vi "Interfaz.vi"() -> ()   [LabVIEW 2025]
uses:
  <vilib>/httpClient/PUTBuffer.vi
  <vilib>/httpClient/LabVIEWHTTPClient.lvlib
panel:
  in  "Ganacias \ny \nSetpoint":T1
  in  "Paro":bool
  out "Error 2":dbl(graph)
  out "Fuera de servicio":bool
  out "Posicion":dbl
  out "Heartbeat":dbl
  out "error\n out":errorcluster
  out "Error":dbl
  # "INSTITUTO POLITECNICO NACIONAL"
  # "Unidad Profesional Interdisciplinaria de Ingeniería\nCampus Zacatecas"
  # "Botones"
  # "Resultados"
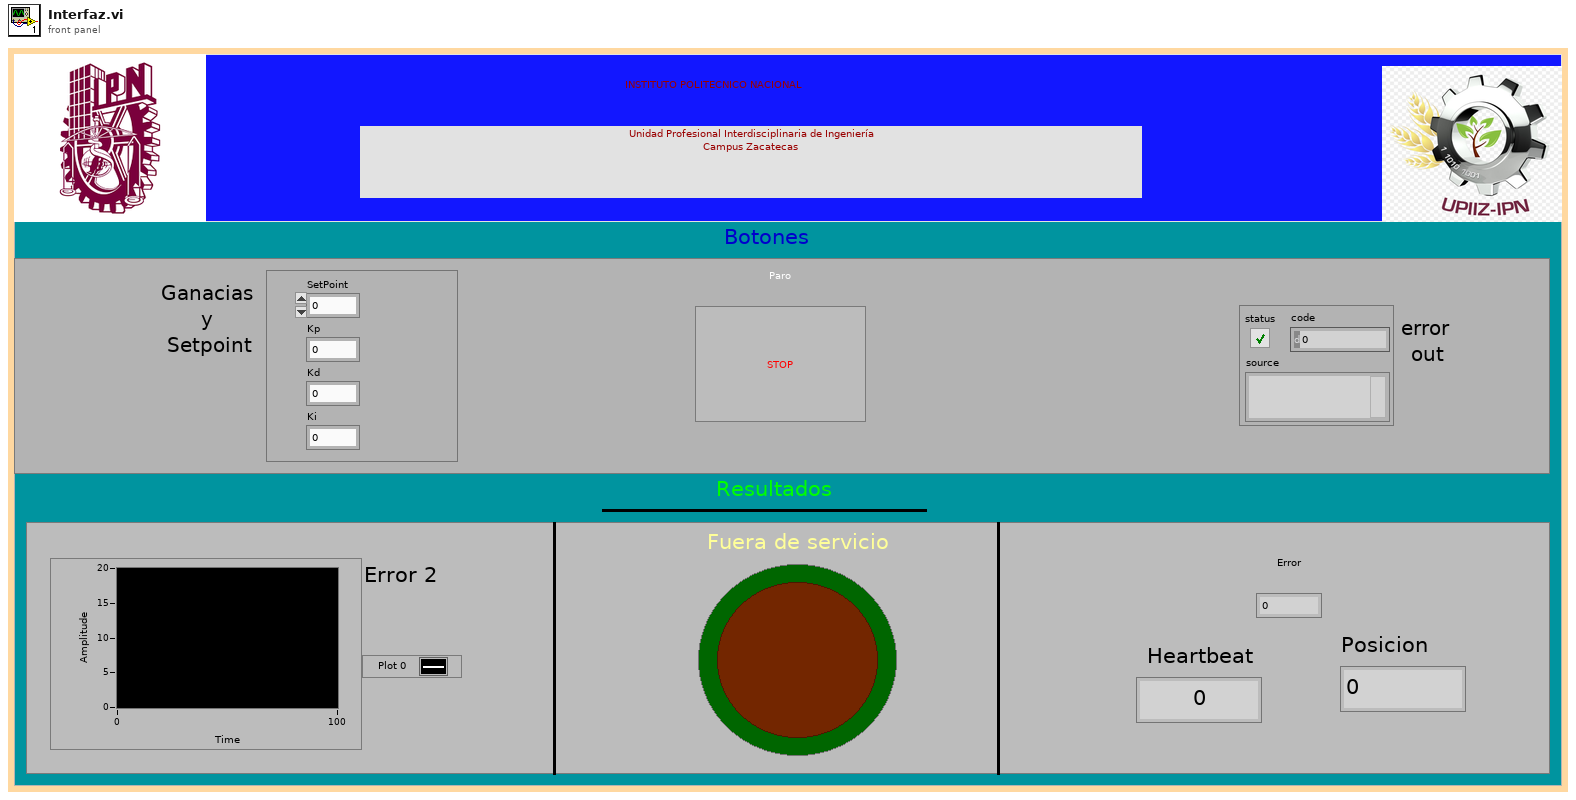
[diagram p1: front panel]
types:
  T1 = cluster{"SetPoint":dbl, "Kp":dbl, "Ki":dbl, "Kd":dbl}
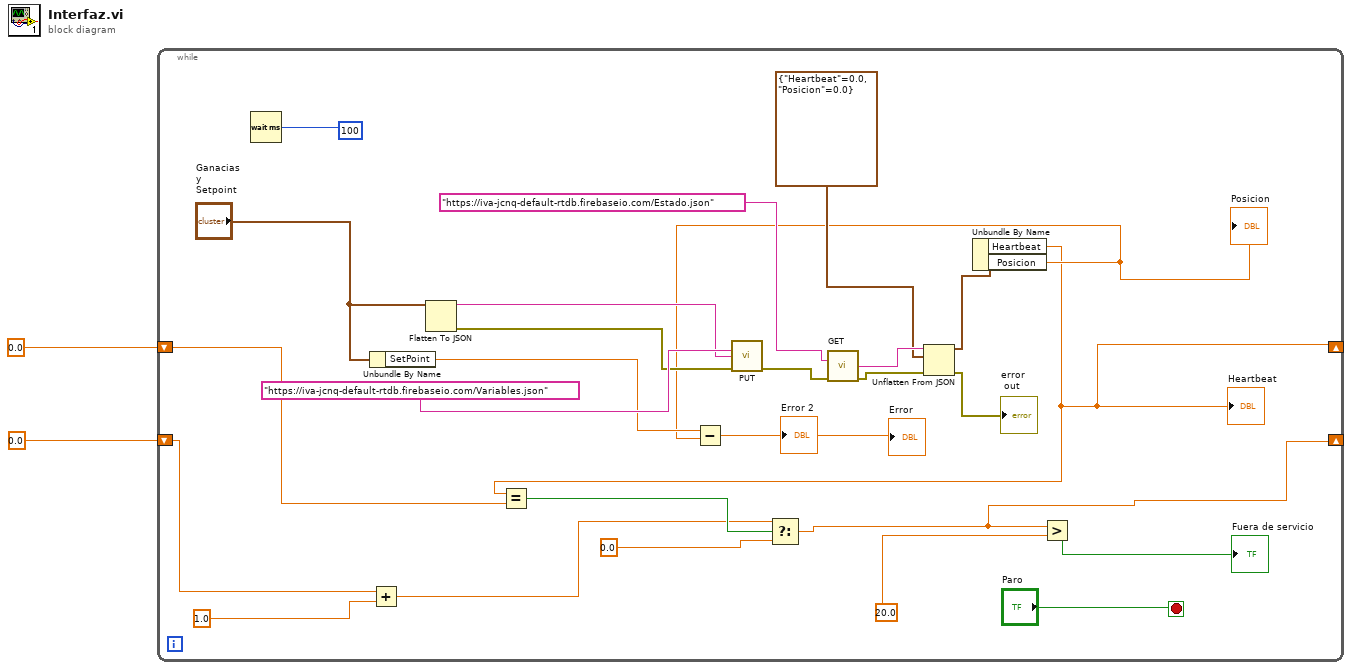
[diagram p0: block diagram]
diagram:
  n1 = while {
    shift-right: [w3] -> _
    shift-left: 0.0 ("x") -> [w17]
    shift-right: [w9] -> _
    shift-left: 0.0 ("x") -> [w14]
    stop <- "Paro" stop-if-true
    n2 = Wait (ms)(milliseconds to wait=u32 100) -> ()  [unwired: 1 out]
    n3 = Unbundle By Name("Ganacias \ny \nSetpoint") -> ("SetPoint"=w19:dbl)
    n4 = Add(x=w14, y=1.0) -> (x+y=w12:dbl)
    n5 = Flatten To JSON(anything="Ganacias \ny \nSetpoint") -> (JSON string=w25:string, 11:w26:errorcluster)  [unwired: 2 in]
    n6 = call-poly <vilib>:"PUT.vi"("url"="https://iva-jcnq-default-rtdb.firebaseio.com/Variables.json", "buffer"=w25, "error in (no error)"=w26) -> ("error out"=w24:errorcluster)  [unwired: 9 in, 3 out]
    n7 = call <vilib>:"GET.vi"("url"="https://iva-jcnq-default-rtdb.firebaseio.com/Estado.json", "error in (no error)"=w24) -> ("body"=w22:string, "error out"=w7:errorcluster)  [unwired: 10 in, 2 out]
    n8 = Unflatten From JSON(JSON string=w22, type and defaults=cluster{"Heartbeat":dbl, "Posicion":dbl} {"Heartbeat"=0.0, "Posicion"=0.0}, error in (no error)=w7) -> (value=w5:cluster{"Heartbeat":dbl, "Posicion":dbl}, error out=→"error\n out":errorcluster)  [unwired: 4 in]
    n9 = Unbundle By Name(w5) -> ("Heartbeat"=w3:dbl, "Posicion"=w4:dbl)
    "Posicion" <- w4
    "Heartbeat" <- w3
    n10 = Equal?(x=w3, y=w17) -> (x = y?=w15:bool)
    n11 = Subtract(x=w19, y=w4) -> (x-y=→"Error 2" →"Error":dbl)
    n12 = Select(t=w12, s=w15, f=0.0) -> (s? t:f=w9:dbl)
    n13 = Greater?(x=w9, y=20.0 ("x")) -> (0:→"Fuera de servicio":bool)
  }
